vi "FPGA Main - 9025.vi"() -> ()   [LabVIEW 2017]
uses:
  Controls/Logging Settings FPGA.ctl
  Controls/Manual Control FPGA.ctl
  <vilib>/rvi/eio/common/nirviEmuTemplateMethod_errors.vi
  <vilib>/rvi/Emulation/niFpgaGetClockAttributes.vi
  <vilib>/rvi/Emulation/niFpgaSctlEmulationGetInTimedLoop.vi
  <vilib>/rvi/Emulation/niFpgaEmulationReportErrorSimple.vi
  <vilib>/rvi/Emulation/niFpgaProcessEmulError.vi
  <vilib>/rvi/interface/RandomDataEmulation/niFpgaRandomDataHandleErrors.vi
  <vilib>/rvi/Emulation/niFpgaCriticalErrorInLSC.vi
  <vilib>/eio/EIONode/EIONode.xnode
  <vilib>/rvi/DataTransferAndStorage/Container/XNode/niFpgaContainer.xnode
  <vilib>/rvi/interface/RandomDataEmulation/nirviRandomDataFpgaReadWriteTemplate.vi
panel:
  out "TC FIFO Timed Out":bool
  in  "High Speed?":bool
  in  "Logging?":bool
  in  "Poll Rate":u32
  out "PS FIFO Timed Out":bool
  out "LC FIFO Timed Out":bool
  in  "Actuator Settings":T1 {"Emergency State" items=["Closed", "Open"]; "Output Port" items=["DIDO/DO0", "DIDO/DO1", "DIDO/DO2", "DIDO/DO3", "DIDO/DO4", "DIDO/DO5", "DIDO/DO6", "DIDO/DO7", "DIDO/DO8", "DIDO/DO9", "DIDO/DO10", "DIDO/DO11", "DIDO/DO12", "DIDO/DO13", "DIDO/DO14", "DIDO/DO15", "PWM/DO0", "PWM/DO1", "PWM/DO2", "PWM/DO3", "PWM/DO4", "PWM/DO5", "PWM/DO6", "PWM/DO7"]; "Unpowered State" items=["Closed", "Opened"]}
  out "FPGA States":T2(ring)
  in  "Manual Mode":bool=TRUE
  in  "Start Automated Sequence":bool
  in  "Emergency Shutdown":bool
  out "Automated Sequence Timer":i32
  in  "Emergency Normally Open/Closed":bool
  out "Emergency Triggered":bool
  in  "Emergency Shutdown Channel":T3(ring)
  in  "Logging Settings":T4
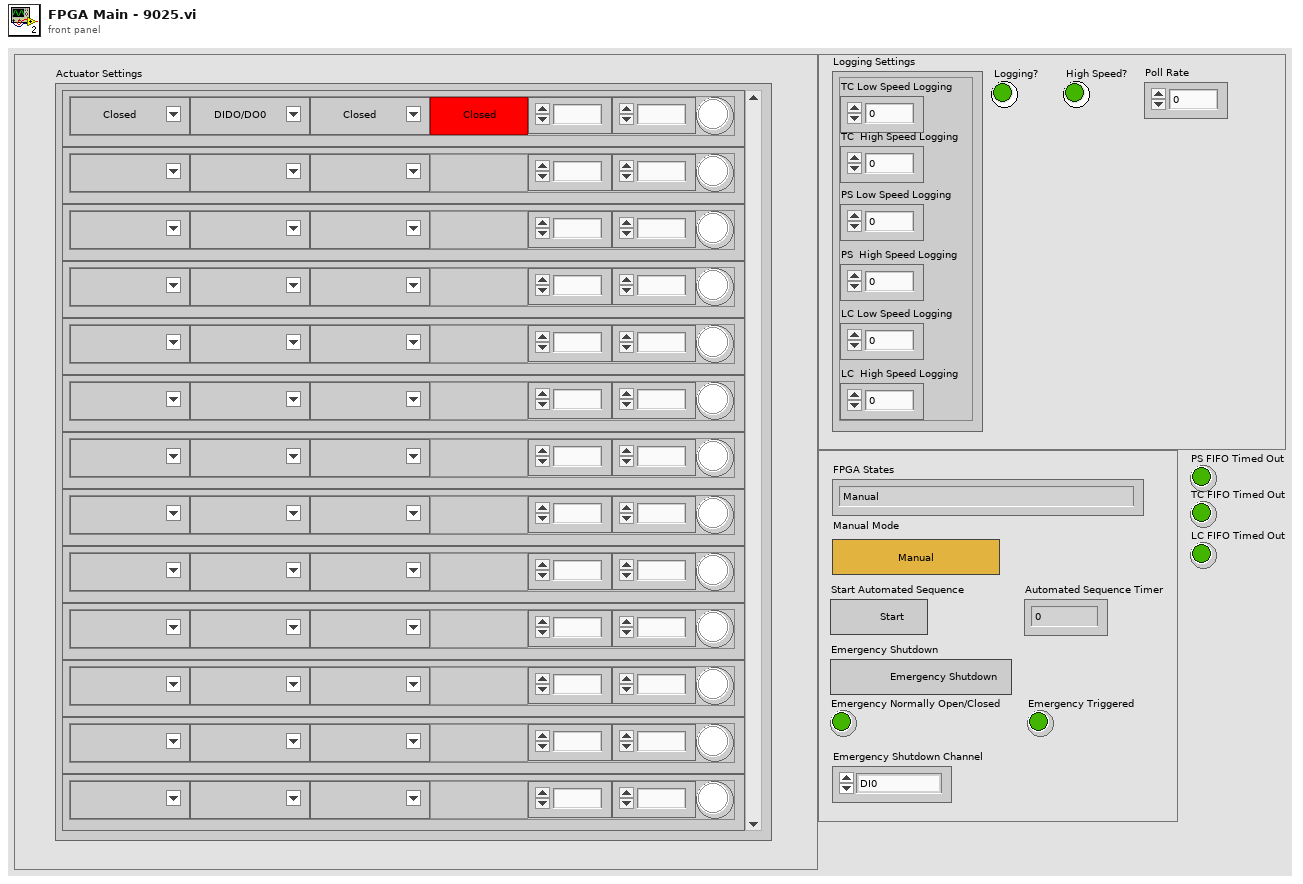
[diagram p1: front panel]
types:
  T1 = typedef "Manual Control FPGA.ctl" = cluster{"Unpowered State":u8, "Output Port":u8, "Emergency State":u8, "Blank Button":bool, "Open Time [ms]":fxp<+/-,18,18>, "Close Time [ms]":fxp<+/-,18,18>, "Active":bool}[]
  T2 = enum16{"Manual", "Standby", "Automated Sequence", "Automated Sequence End", "Emergency"}
  T3 = enum16{"DI0", "DI1", "DI2", "DI3", "DI4", "DI5", "DI7", "DI6", "DI8", "DI9", "DI10", "DI11", "DI12", "DI13", "DI14", "DI15"}
  T4 = typedef "Logging Settings FPGA.ctl" = cluster{"TC Low Speed Logging":u32, "TC  High Speed Logging":u32, "PS Low Speed Logging":u32, "PS  High Speed Logging":u32, "LC Low Speed Logging":u32, "LC  High Speed Logging":u32}
  T5 = cluster{"Unpowered State":u8, "Output Port":u8, "Emergency State":u8, "Blank Button":bool, "Open Time [ms]":fxp<+/-,18,18>, "Close Time [ms]":fxp<+/-,18,18>, "Active":bool}
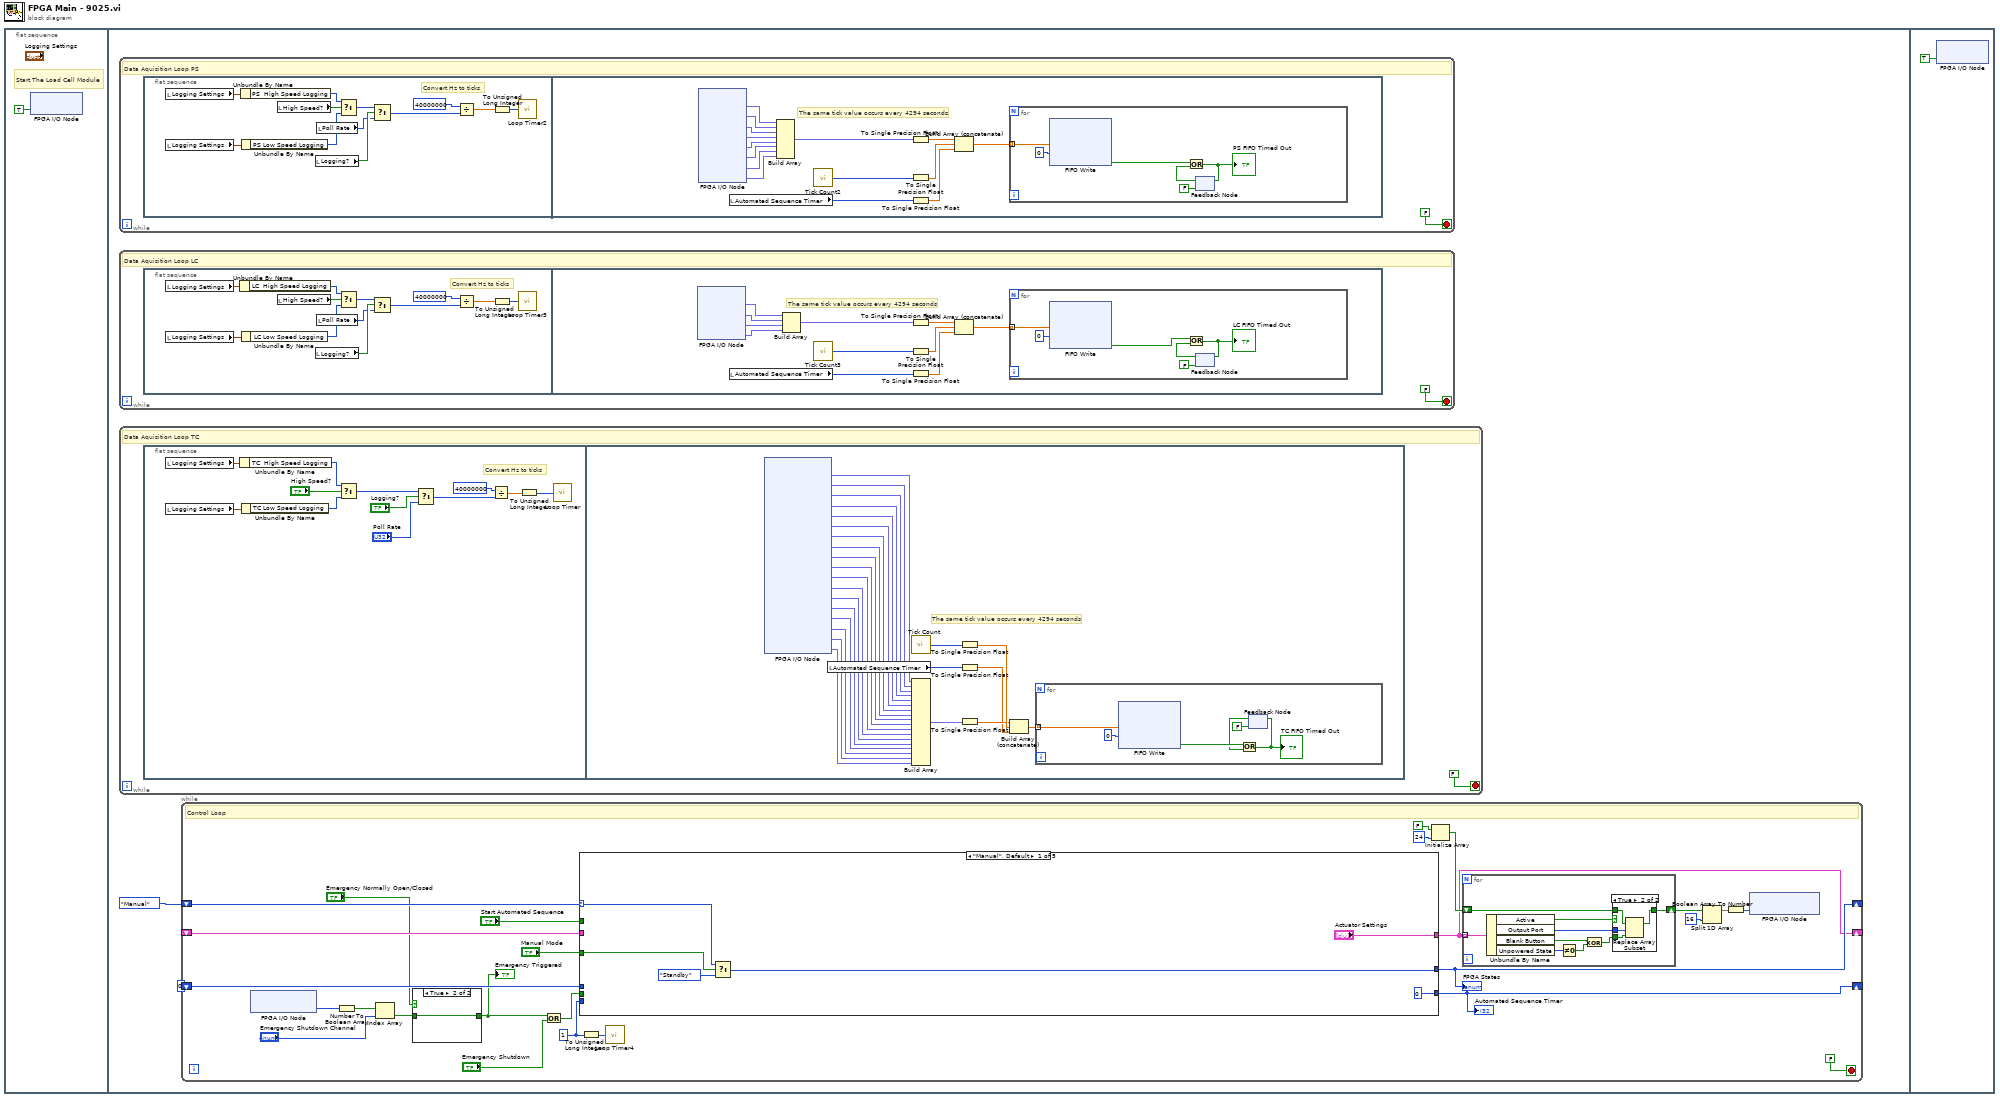
[diagram p0: block diagram]
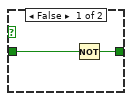
[diagram p2: hidden frame]
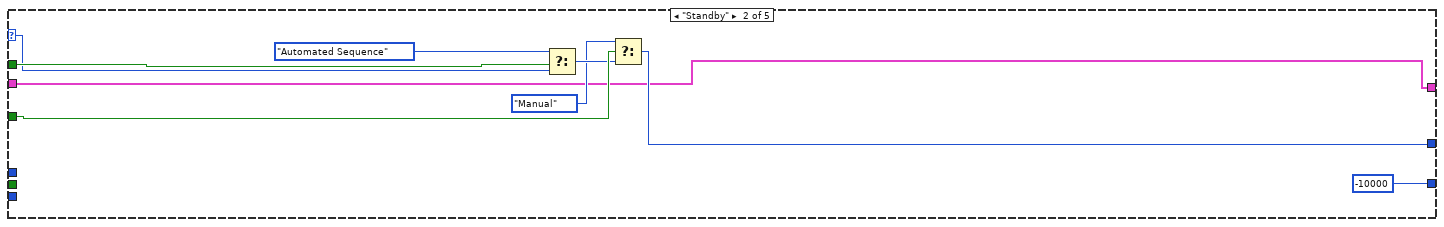
[diagram p4: hidden frame]
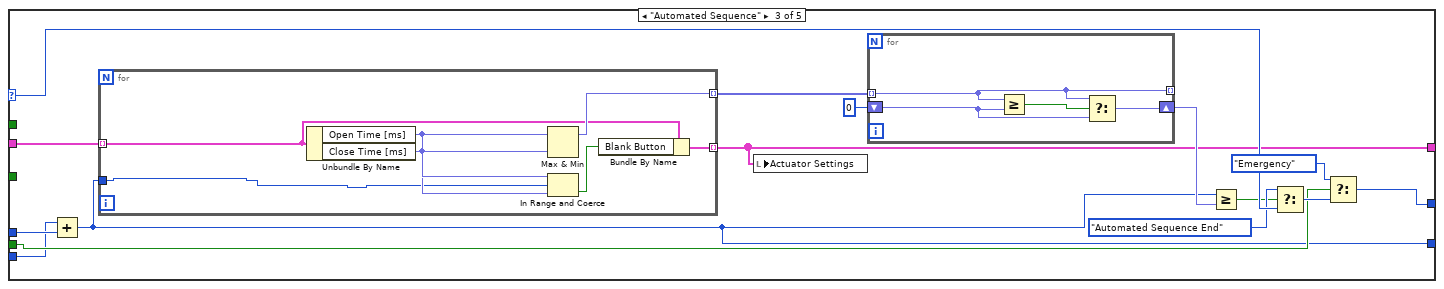
[diagram p5: hidden frame]
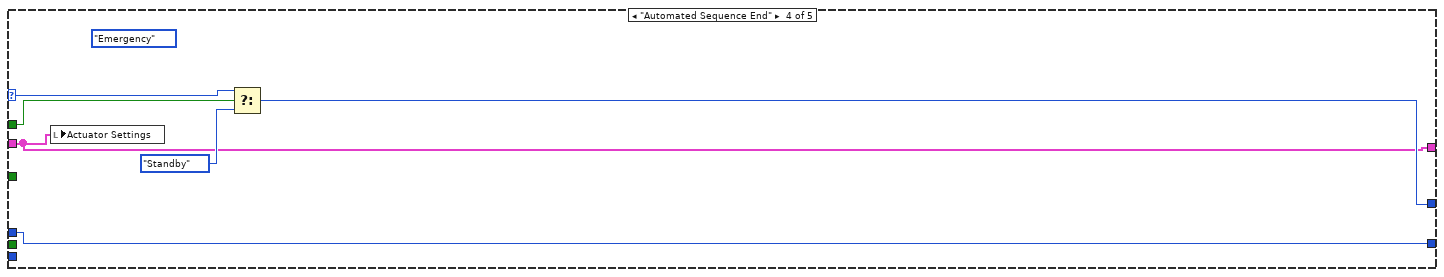
[diagram p6: hidden frame]
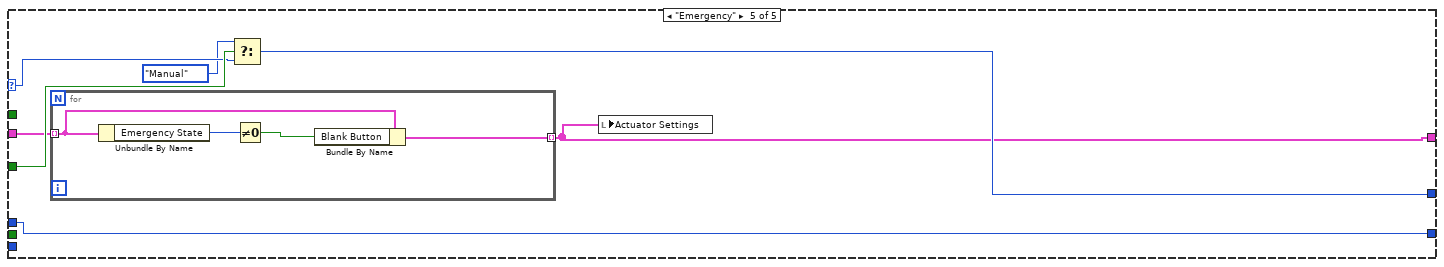
[diagram p7: hidden frame]
diagram:
  n1 = flat-sequence {
    frame #0 {
      # "Start The Load Cell Module"
      n2 = xnode "FPGA I/O Node"("LC/Start"=TRUE) -> ()  [unwired: 1 in, 1 out]
    }
    frame #1 {
      n3 = while {
        stop <- FALSE stop-if-true
        # "Data Aquisition Loop PS"
        n4 = flat-sequence {
          frame #0 {
            # "Convert Hz to ticks"
            n5 = local read "Logging Settings"() -> (w142:T4)
            n6 = local read "Logging Settings"() -> (w140:T4)
            n7 = Unbundle By Name(w142) -> ("PS  High Speed Logging"=w137:u32)
            n8 = Unbundle By Name(w140) -> ("PS Low Speed Logging"=w136:u32)
            n9 = local read "High Speed?"() -> (w141:bool)
            n10 = local read "Logging?"() -> (w139:bool)
            n11 = local read "Poll Rate"() -> (w138:u32)
            n12 = Select(t=w137, s=w141, f=w136) -> (s? t:f=w144:u32)
            n13 = Select(t=w144, s=w139, f=w138) -> (s? t:f=w143:u32)
            n14 = Divide(x=u32 40000000, y=w143) -> (x/y=w146:sgl)
            n15 = To Unsigned Long Integer(number=w146) -> (unsigned 32bit integer=w145:u32)
            n16 = call "Loop Timer2"("Count(Ticks)"=w145) -> ()  [unwired: 1 out]
          }
          frame #1 {
            # "The same tick value occurs every 4294 seconds"
            n17 = xnode "FPGA I/O Node"() -> ("PS/AI0"=w162:fxp<+/-,21,-4>, "PS/AI1"=w156:fxp<+/-,21,-4>, "PS/AI2"=w155:fxp<+/-,21,-4>, "PS/AI3"=w154:fxp<+/-,21,-4>, "PS/AI4"=w153:fxp<+/-,21,-4>, "PS/AI5"=w152:fxp<+/-,21,-4>, "PS/AI6"=w151:fxp<+/-,21,-4>, "PS/AI7"=w150:fxp<+/-,21,-4>)  [unwired: 8 in, 8 out]
            n18 = local read "Automated Sequence Timer"() -> (w149:i32)
            n19 = Build Array(w162, w156, w155, w154, w153, w152, w151, w150) -> (w161:fxp<+/-,21,-4>[])
            n20 = call "Tick Count2"() -> ("Tick Count(uSec)"=w159:u32)
            n21 = To Single Precision Float(number=w161) -> (single precision float=w157:sgl[])
            n22 = To Single Precision Float(number=w159) -> (single precision float=w158:sgl)
            n23 = To Single Precision Float(number=w149) -> (single precision float=w148:sgl)
            n24 = Build Array (concatenate)(w157, w158, w148) -> (w160:sgl[])
            n25 = for {
              tunnel: w160 -> [w168] mode=indexing
              n26 = xnode ("FIFO Write")("Element"=w168, "Timeout"=0) -> ("Timed Out?"=w166:bool)  [unwired: 1 in, 1 out]
              n27 = feedback #1(FALSE ("Timed Out?")) -> (w163:bool)
              n28 = Or(x=w166, y=w163) -> (x .or. y?=w164:bool)
              "PS FIFO Timed Out" <- w164
              n29 = feedback-in #1(w164) -> ()
            }
          }
        }
      }
      n30 = while {
        stop <- FALSE stop-if-true
        # "Data Aquisition Loop LC"
        n31 = flat-sequence {
          frame #0 {
            # "Convert Hz to ticks"
            n32 = local read "Logging Settings"() -> (w113:T4)
            n33 = local read "Logging Settings"() -> (w111:T4)
            n34 = Unbundle By Name(w113) -> ("LC  High Speed Logging"=w107:u32)
            n35 = Unbundle By Name(w111) -> ("LC Low Speed Logging"=w108:u32)
            n36 = local read "High Speed?"() -> (w112:bool)
            n37 = local read "Logging?"() -> (w110:bool)
            n38 = local read "Poll Rate"() -> (w109:u32)
            n39 = Select(t=w107, s=w112, f=w108) -> (s? t:f=w106:u32)
            n40 = Select(t=w106, s=w110, f=w109) -> (s? t:f=w114:u32)
            n41 = Divide(x=u32 40000000, y=w114) -> (x/y=w116:sgl)
            n42 = To Unsigned Long Integer(number=w116) -> (unsigned 32bit integer=w115:u32)
            n43 = call "Loop Timer3"("Count(Ticks)"=w115) -> ()  [unwired: 1 out]
          }
          frame #1 {
            # "The same tick value occurs every 4294 seconds"
            n44 = xnode "FPGA I/O Node"() -> ("LC/AI0"=w128:fxp<+/-,24,-4>, "LC/AI1"=w122:fxp<+/-,24,-4>, "LC/AI2"=w121:fxp<+/-,24,-4>, "LC/AI3"=w120:fxp<+/-,24,-4>)  [unwired: 4 in, 4 out]
            n45 = local read "Automated Sequence Timer"() -> (w119:i32)
            n46 = Build Array(w128, w122, w121, w120) -> (w127:fxp<+/-,24,-4>[])
            n47 = call "Tick Count3"() -> ("Tick Count(uSec)"=w125:u32)
            n48 = To Single Precision Float(number=w127) -> (single precision float=w123:sgl[])
            n49 = To Single Precision Float(number=w125) -> (single precision float=w124:sgl)
            n50 = To Single Precision Float(number=w119) -> (single precision float=w118:sgl)
            n51 = Build Array (concatenate)(w123, w124, w118) -> (w126:sgl[])
            n52 = for {
              tunnel: w126 -> [w134] mode=indexing
              n53 = xnode ("FIFO Write")("Element"=w134, "Timeout"=0) -> ("Timed Out?"=w132:bool)  [unwired: 1 in, 1 out]
              n54 = feedback #2(FALSE ("Timed Out?")) -> (w129:bool)
              n55 = Or(x=w132, y=w129) -> (x .or. y?=w130:bool)
              "LC FIFO Timed Out" <- w130
              n56 = feedback-in #2(w130) -> ()
            }
          }
        }
      }
      n57 = while {
        stop <- FALSE stop-if-true
        # "Data Aquisition Loop TC"
        n58 = flat-sequence {
          frame #0 {
            # "Convert Hz to ticks"
            n59 = local read "Logging Settings"() -> (w173:T4)
            n60 = local read "Logging Settings"() -> (w171:T4)
            n61 = Unbundle By Name(w173) -> ("TC  High Speed Logging"=w172:u32)
            n62 = Unbundle By Name(w171) -> ("TC Low Speed Logging"=w170:u32)
            n63 = Select(t=w172, s="High Speed?", f=w170) -> (s? t:f=w176:u32)
            n64 = Select(t=w176, s="Logging?", f="Poll Rate") -> (s? t:f=w174:u32)
            n65 = Divide(x=u32 40000000, y=w174) -> (x/y=w179:sgl)
            n66 = To Unsigned Long Integer(number=w179) -> (unsigned 32bit integer=w178:u32)
            n67 = call "Loop Timer"("Count(Ticks)"=w178) -> ()  [unwired: 1 out]
          }
          frame #1 {
            # "The same tick value occurs every 4294 seconds"
            n68 = xnode "FPGA I/O Node"() -> ("TC/TC0"=w206:fxp<+/-,24,-2>, "TC/TC1"=w200:fxp<+/-,24,-2>, "TC/TC2"=w199:fxp<+/-,24,-2>, "TC/TC3"=w198:fxp<+/-,24,-2>, "TC/TC4"=w197:fxp<+/-,24,-2>, "TC/TC5"=w196:fxp<+/-,24,-2>, "TC/TC6"=w195:fxp<+/-,24,-2>, "TC/TC7"=w194:fxp<+/-,24,-2>, "TC/TC8"=w193:fxp<+/-,24,-2>, "TC/TC9"=w192:fxp<+/-,24,-2>, "TC/TC10"=w191:fxp<+/-,24,-2>, "TC/TC11"=w190:fxp<+/-,24,-2>, "TC/TC12"=w189:fxp<+/-,24,-2>, "TC/TC13"=w188:fxp<+/-,24,-2>, "TC/TC14"=w187:fxp<+/-,24,-2>, "TC/TC15"=w186:fxp<+/-,24,-2>, "TC/Autozero"=w185:fxp<+/-,24,-2>, "TC/CJC"=w184:fxp<+/-,24,-2>)  [unwired: 18 in, 18 out]
            n69 = local read "Automated Sequence Timer"() -> (w183:i32)
            n70 = call "Tick Count"() -> ("Tick Count(uSec)"=w203:u32)
            n71 = Build Array(w206, w200, w199, w198, w197, w196, w195, w194, w193, w192, w191, w190, w189, w188, w187, w186, w185, w184) -> (w205:fxp<+/-,24,-2>[])
            n72 = To Single Precision Float(number=w203) -> (single precision float=w202:sgl)
            n73 = To Single Precision Float(number=w183) -> (single precision float=w182:sgl)
            n74 = To Single Precision Float(number=w205) -> (single precision float=w201:sgl[])
            n75 = Build Array (concatenate)(w201, w202, w182) -> (w204:sgl[])
            n76 = for {
              tunnel: w204 -> [w212] mode=indexing
              n77 = xnode ("FIFO Write")("Element"=w212, "Timeout"=0) -> ("Timed Out?"=w210:bool)  [unwired: 1 in, 1 out]
              n78 = feedback #3(FALSE ("Timed Out?")) -> (w207:bool)
              n79 = Or(x=w210, y=w207) -> (x .or. y?=w208:bool)
              "TC FIFO Timed Out" <- w208
              n80 = feedback-in #3(w208) -> ()
            }
          }
        }
      }
      n81 = while {
        shift-right: [w28] -> _
        shift-left: T2."Manual" ("FPGA States") -> [w29]
        shift-right: [w13] -> _
        shift-left: _ -> [w21]
        shift-right: [w24] -> _
        shift-left: 0 -> [w23]
        stop <- FALSE stop-if-true
        w5 = 1 ("Count(mSec)")
        # "Control Loop"
        n82 = xnode "FPGA I/O Node"() -> ("DIDO/DI15:0"=w11:u16)  [unwired: 1 in, 1 out]
        n83 = Number To Boolean Array(number=w11) -> (Boolean array=w8:bool[])
        n84 = Index Array(array=w8, index="Emergency Shutdown Channel") -> (element=w6:bool)
        n85 = case shown="True" "Emergency Normally Open/Closed" {
          tunnel: w6 -> [w31 w32]
          tunnel: [w30 w32] -> w10
          frame False {
            n86 = Not(x=w31) -> (.not. x?=w30:bool)
          }
          frame True {
          }
        }
        "Emergency Triggered" <- w10
        n87 = Or(x=w10, y="Emergency Shutdown") -> (x .or. y?=w12:bool)
        n88 = case shown="\"Manual\", Default" w29 {
          selector: w29 -> [w52 w60 w74 w91 w98]
          tunnel: [w49 w55 w75 w89 w96] -> w28
          tunnel: w12 -> [_ _ w71 _ _]
          tunnel: "Start Automated Sequence" -> [_ w61 _ w92 _]
          tunnel: "Manual Mode" -> [w50 w58 _ _ w99]
          tunnel: [0 -10000 w64 w93 w100] -> w24
          tunnel: w23 -> [_ _ w70 w93 w100]
          tunnel: w5 -> [_ _ w69 _ _]
          tunnel: ["Actuator Settings" w53 w63 w88 w94] -> w13
          tunnel: w21 -> [_ w53 w65 w88 w95]
          frame "Manual", Default {
            n89 = Select(t=w52, s=w50, f=T2."Standby") -> (s? t:f=w49:T2)
          }
          frame "Standby" {
            n90 = Select(t=T2."Automated Sequence", s=w61, f=w60) -> (s? t:f=w57:T2)
            n91 = Select(t=T2."Manual", s=w58, f=w57) -> (s? t:f=w55:T2)
          }
          frame "Automated Sequence" {
            n92 = Add(x=w69, y=w70) -> (x+y=w64:i32)
            n93 = for {
              tunnel: w65 -> [w79] mode=indexing
              tunnel: [w83] -> w66 mode=indexing
              tunnel: w64 -> [w77]
              tunnel: [w78] -> w63 mode=indexing
              n94 = Unbundle By Name(w79) -> ("Open Time [ms]"=w81:fxp<+/-,18,18>, "Close Time [ms]"=w82:fxp<+/-,18,18>)
              n95 = Max & Min(x=w81, y=w82) -> (max(x,y)=w83:fxp<+/-,18,18>)  [unwired: 1 out]
              n96 = In Range and Coerce(upper limit=w82, x=w77, lower limit=w81) -> (In Range?=w80:bool)  [unwired: 1 out]
              n97 = Bundle By Name(cluster=w79, "Blank Button"=w80) -> (w78:T5)
            }
            n98 = local write "Actuator Settings"(w63) -> ()
            n99 = for {
              tunnel: [w84] -> _ mode=indexing
              shift-right: [w87] -> w67
              shift-left: 0 ("y") -> [w85]
              tunnel: w66 -> [w84] mode=indexing
              n100 = Greater Or Equal?(x=w84, y=w85) -> (x >= y?=w86:bool)
              n101 = Select(t=w84, s=w86, f=w85) -> (s? t:f=w87:fxp<+/-,32,32>)
            }
            n102 = Greater Or Equal?(x=w64, y=w67) -> (x >= y?=w62:bool)
            n103 = Select(t=T2."Automated Sequence End", s=w62, f=w74) -> (s? t:f=w72:T2)
            n104 = Select(t=T2."Emergency", s=w71, f=w72) -> (s? t:f=w75:T2)
          }
          frame "Automated Sequence End" {
            (unwired) T2."Emergency" ("t")
            n105 = local write "Actuator Settings"(w88) -> ()
            n106 = Select(t=w91, s=w92, f=T2."Standby" ("FPGA States")) -> (s? t:f=w89:T2)
          }
          frame "Emergency" {
            n107 = for {
              tunnel: w95 -> [w104] mode=indexing
              tunnel: [w101] -> w94 mode=indexing
              n108 = Unbundle By Name(w104) -> ("Emergency State"=w102:u8)
              n109 = Not Equal To 0?(x=w102) -> (x != 0?=w103:bool)
              n110 = Bundle By Name(cluster=w104, "Blank Button"=w103) -> (w101:T5)
            }
            n111 = Select(t=T2."Manual", s=w99, f=w98) -> (s? t:f=w96:T2)
            n112 = local write "Actuator Settings"(w94) -> ()
          }
        }
        "FPGA States" <- w28
        "Automated Sequence Timer" <- w24
        n113 = To Unsigned Long Integer(number=w5) -> (unsigned 32bit integer=w4:u32)
        n114 = call "Loop Timer4"("Count(mSec)"=w4) -> ()  [unwired: 1 out]
        n115 = Initialize Array(FALSE, 24 ("dimension size")) -> (w19:bool[])
        n116 = for {
          tunnel: w13 -> [w41] mode=indexing
          shift-right: [w36] -> w18
          shift-left: w19 -> [w37]
          n117 = Unbundle By Name(w41) -> ("Active"=w33:bool, "Output Port"=w35:u8, "Blank Button"=w40:bool, "Unpowered State"=w39:u8)
          n118 = Not Equal To 0?(x=w39) -> (x != 0?=w38:bool)
          n119 = Exclusive Or(1:w38, 2:w40) -> (0:w34:bool)
          n120 = case shown="True" w33 {
            tunnel: w37 -> [w42 w46]
            tunnel: [w42 w45] -> w36
            tunnel: w35 -> [_ w44]
            tunnel: w34 -> [_ w43]
            frame False {
            }
            frame True {
              n121 = Replace Array Subset(array=w46, new element=w43, index=w44) -> (w45:bool[])
            }
          }
        }
        n122 = Split 1D Array(array=w18, index=16) -> (first subarray=w15:bool[])  [unwired: 1 out]
        n123 = Boolean Array To Number(Boolean array=w15) -> (number=w16:u16)
        n124 = xnode "FPGA I/O Node"("DIDO/DO15:0"=w16) -> ()  [unwired: 1 in, 1 out]
      }
    }
    frame #2 {
      n125 = xnode "FPGA I/O Node"("LC/Stop"=TRUE ("LC/Start")) -> ()  [unwired: 1 in, 1 out]
    }
  }
